vi "Init.vi"(7 "Sender":refnum<class "Sender.lvclass">, 9 "Error":errorcluster, 10 "Actor":refnum<class "Actor.lvclass">) -> (3 "Has Destroyed Msg out":refnum<class "Has Destroyed Msg.lvclass">)   [LabVIEW 2020, in "jettl.lvlib" / "Has Destroyed Msg.lvlib" / "Has Destroyed Msg.lvclass"]
uses:
  Has Destroyed Msg.lvclass
  Actor/Actor/Actor.lvclass
  Sender/Sender/Sender.lvclass
  Has Destroyed Msg.lvclass/Has Destroyed Msg.ctl
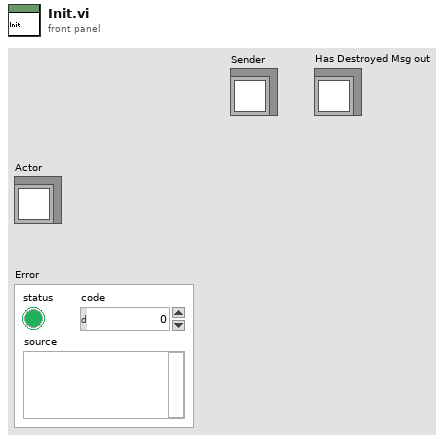
[diagram p1: front panel]
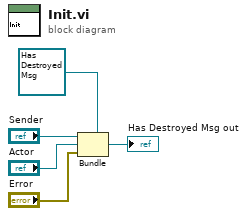
[diagram p0: block diagram]
diagram:
  n1 = Bundle "Bundle"(cluster=refnum<class "Has Destroyed Msg.lvclass"> refnum ("Last Ack Creator Queue Msg Strategy out"), "Sender", "Actor", "Error") -> (→"Has Destroyed Msg out":refnum<class "Has Destroyed Msg.lvclass">)
